vi "Check Scan Position.vi"() -> ()   [LabVIEW 2019]
panel:
  in  "stop":bool
  out "XY Graph":cluster{u32[], dbl[]}(graph)
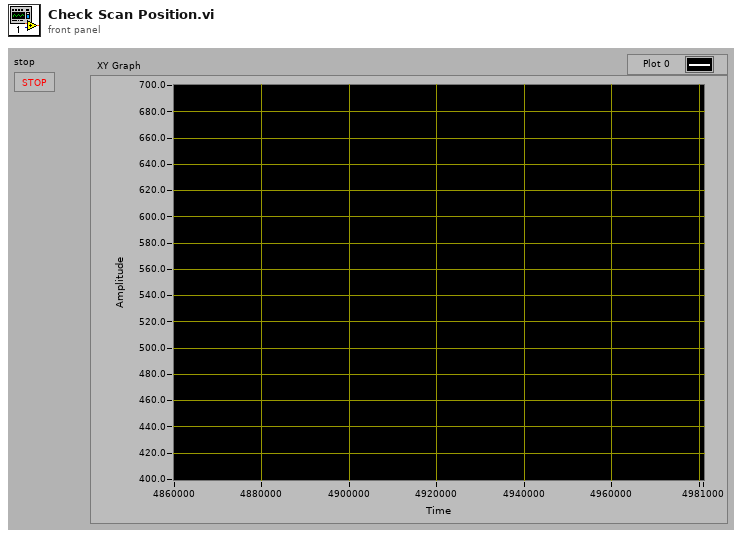
[diagram p1: front panel]
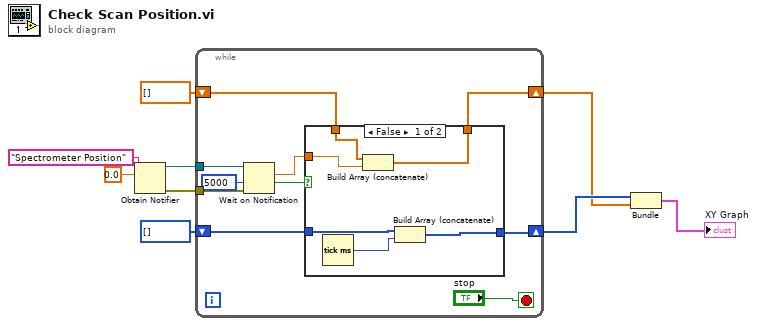
[diagram p0: block diagram]
diagram:
  n1 = Obtain Notifier(name (unnamed)="Spectrometer Position", notification data type=0.0 ("Speed")) -> (notifier out=w7:refnum<notifier>, error out=w6:errorcluster)  [unwired: 2 in, 1 out]
  n2 = while {
    tunnel: w7 -> [w19]
    tunnel: w6 -> [w18]
    shift-right: [w16] -> w3
    shift-left: dbl[] [] -> [w15]
    shift-right: [w13] -> w4
    shift-left: u32[] [] -> [w14]
    stop <- "stop" stop-if-true
    n3 = Wait on Notification(notifier=w19, timeout in ms (-1)=5000, error in (no error)=w18) -> (notification=w17:dbl, timed out?=w12:bool)  [unwired: 1 in, 2 out]
    n4 = case shown="False" w12 {
      tunnel: w17 -> [w25 _]
      tunnel: [w24 w26] -> w16
      tunnel: w15 -> [w23 w26]
      tunnel: w14 -> [w22 w27]
      tunnel: [w21 w27] -> w13
      frame False {
        n5 = Tick Count (ms)() -> (millisecond timer value=w20:u32)
        n6 = Build Array (concatenate)(w23, w25) -> (w24:dbl[])
        n7 = Build Array (concatenate)(w22, w20) -> (w21:u32[])
      }
      frame True {
      }
    }
  }
  n8 = Bundle(w4, w3) -> (→"XY Graph":cluster{u32[], dbl[]})  [unwired: 1 in]
